vi "Main.vi"() -> ()   [LabVIEW 2021]
uses:
  <vilib>/httpClient/LabVIEWHTTPClient.lvlib
  <vilib>/wsapi/NI_WebServices.lvlib
panel:
  out "2D Picture":picture
  in  "Get Image":bool
  in  "Get Status":bool
  in  "Get State":bool
  out "Body":string
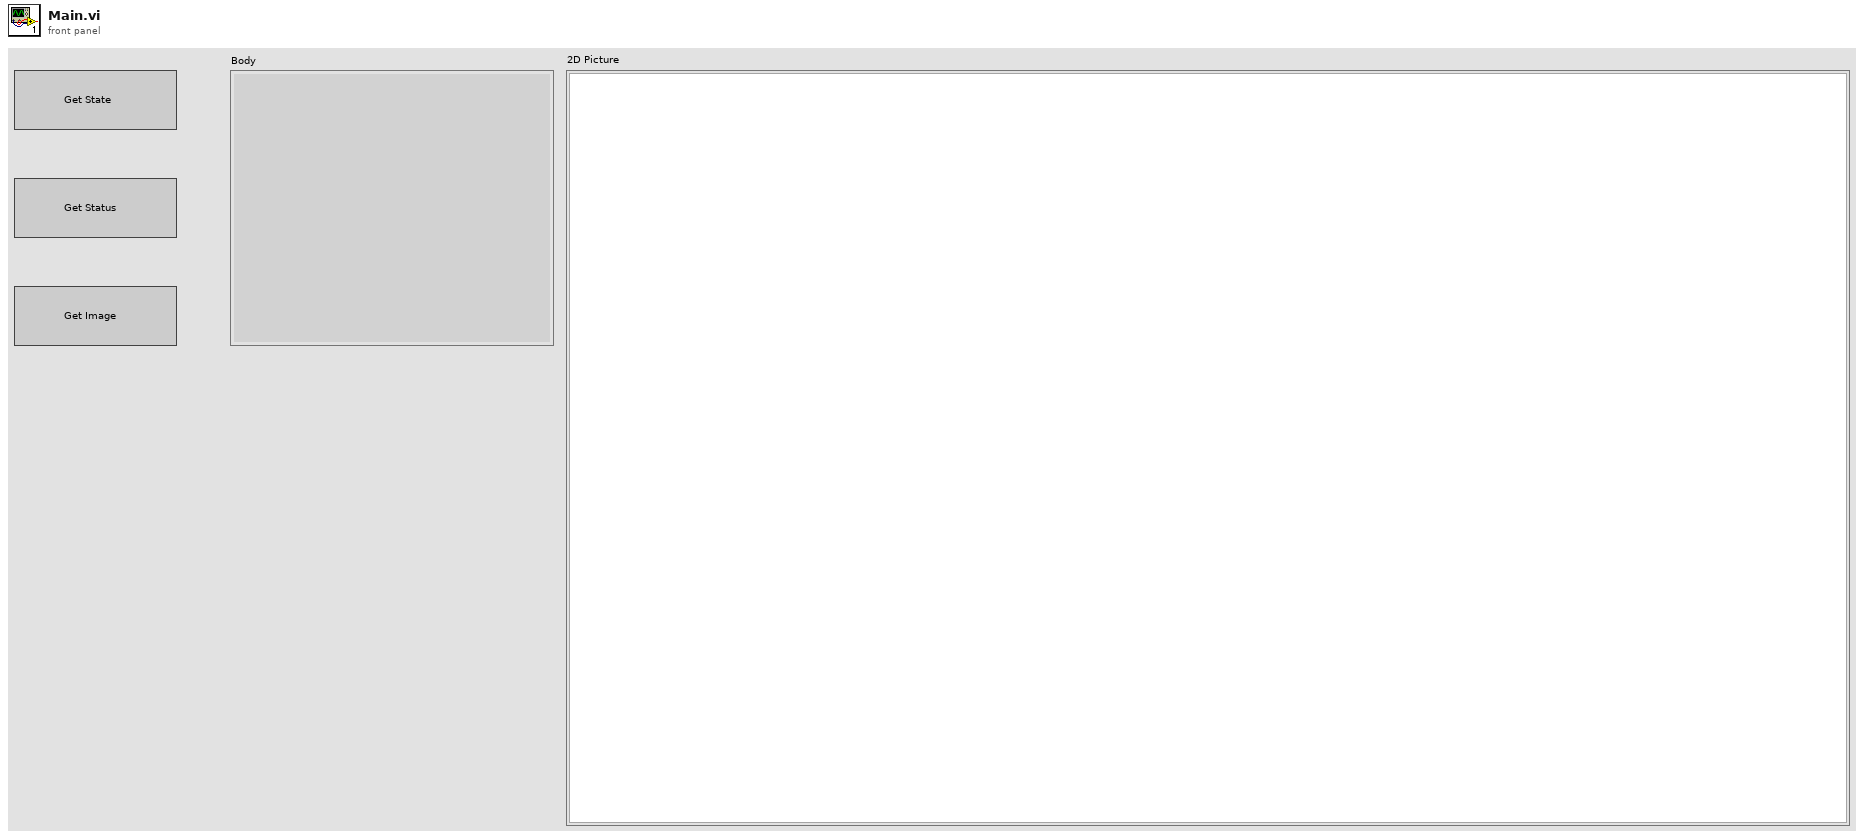
[diagram p1: front panel]
types:
  T1 = typedef "imagedata.ctl" = cluster{"image type":i32, "image depth":i32, "image":u8[], "mask":u8[], "colors":u32[], "Rectangle":cluster{"left":i16, "top":i16, "right":i16, "bottom":i16}}
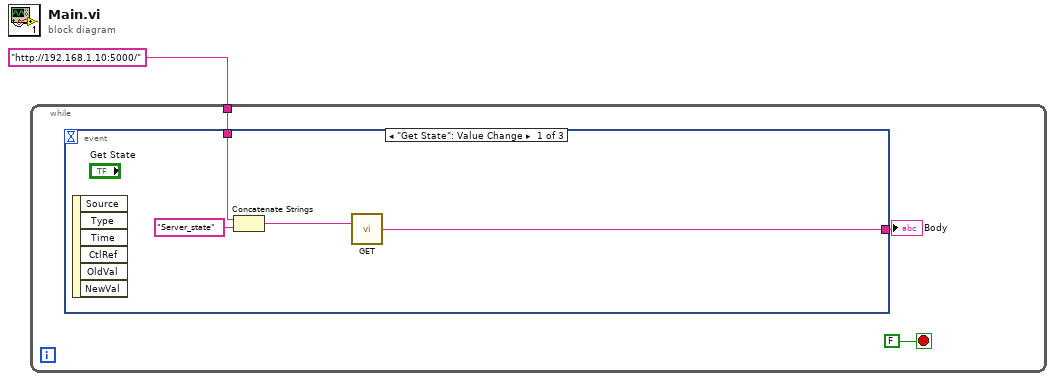
[diagram p0: block diagram]
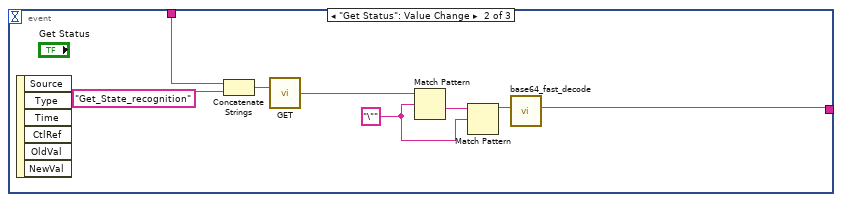
[diagram p2: hidden frame]
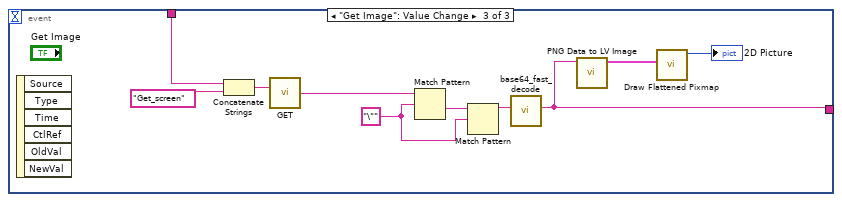
[diagram p3: hidden frame]
diagram:
  n1 = while {
    tunnel: "http://192.168.1.10:5000/" ("url") -> [w4]
    stop <- FALSE stop-if-true
    n2 = event shown="[0] \"Get State\": Value Change" {
      selector: _ -> [_ _ _]
      dyn-events: _ -> [_ _ _]
      timeout: _ -> [_ _ _]
      tunnel: [w5 w11 w19] -> w2
      tunnel: w4 -> [w7 w14 w24]
      event "Get State": Value Change {
        n3 = event-data() -> ()  [unwired: 1 in, 6 out]
        n4 = Concatenate Strings(w7, "Server_state" ("string")) -> (w8:string)
        n5 = call <vilib>:"GET.vi"("url"=w8) -> ("body"=w5:string)  [unwired: 11 in, 3 out]
      }
      event "Get Status": Value Change {
        w9 = "\"" ("regular expression")
        n6 = event-data() -> ()  [unwired: 1 in, 6 out]
        n7 = Concatenate Strings(w14, "Get_State_recognition" ("string")) -> (w16:string)
        n8 = call <vilib>:"GET.vi"("url"=w16) -> ("body"=w10:string)  [unwired: 11 in, 3 out]
        n9 = Match Pattern(string=w10, regular expression=w9) -> (after substring=w13:string)  [unwired: 1 in, 3 out]
        n10 = Match Pattern(string=w13, regular expression=w9) -> (before substring=w12:string)  [unwired: 1 in, 3 out]
        n11 = call "base64_fast_decode.vi"("string in (base64-encoded)"=w12) -> ("string out (decoded)"=w11:string)  [unwired: 9 in, 1 out]
      }
      event "Get Image": Value Change {
        w20 = "\"" ("regular expression")
        n12 = event-data() -> ()  [unwired: 1 in, 6 out]
        n13 = Concatenate Strings(w24, "Get_screen" ("string")) -> (w26:string)
        n14 = call <vilib>:"GET.vi"("url"=w26) -> ("body"=w21:string)  [unwired: 11 in, 3 out]
        n15 = Match Pattern(string=w21, regular expression=w20) -> (after substring=w23:string)  [unwired: 1 in, 3 out]
        n16 = Match Pattern(string=w23, regular expression=w20) -> (before substring=w22:string)  [unwired: 1 in, 3 out]
        n17 = call "base64_fast_decode.vi"("string in (base64-encoded)"=w22) -> ("string out (decoded)"=w19:string)  [unwired: 9 in, 1 out]
        n18 = call <vilib>:"PNG Data to LV Image.vi"("png data"=w19) -> ("image data"=w18:T1)  [unwired: 9 in, 1 out]
        n19 = call <vilib>:"Draw Flattened Pixmap.vi"("image data"=w18) -> ("new picture"=→"2D Picture":picture)  [unwired: 8 in]
      }
    }
    "Body" <- w2
  }
